vi "RSZVB Get Generator Attenuator Mode.vi"(8 "error in (no error)":errorcluster {"code" format="%.0x"}, 9 "Port (1)":i32=1, 10 "Channel (1)":i32=1, 11 "VISA session":refnum<visa-resource-name>) -> (0 "error out":errorcluster {"code" format="%.0x"}, 1 "Attenuation Mode":i32, 3 "dup VISA session":refnum<visa-resource-name>)   [LabVIEW 2011]
doc: "This VI returns the mode of the attenuation factor for the generated wave at test port no. <Pt>. \n\nNote(s):\n\n(1) This VI can be used only with R&S ZVA and ZVB instruments.\n\nRemote-control command(s):\nSOURce<Ch>:POWer<Pt>:ATTenuation:MODE?"
uses:
  _utility/RSZVB Global Data.vi
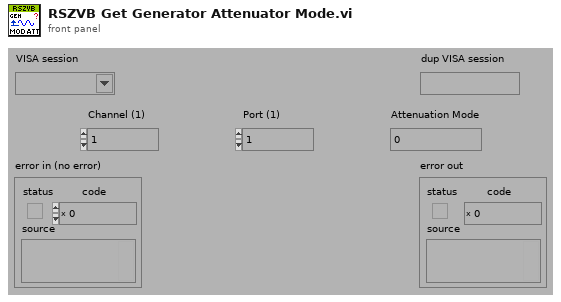
[diagram p1: front panel]
types:
  T1 = cluster{"Error Checking (T: On)":bool, "Installed Options":string[], "Data Valid?":bool, "Ports":i32, "Model":string[], "Option Checking (T: On)":bool}[]
  T2 = cluster{"Error Checking (T: On)":bool, "Installed Options":string[], "Data Valid?":bool, "Ports":i32, "Model":string[], "Option Checking (T: On)":bool}
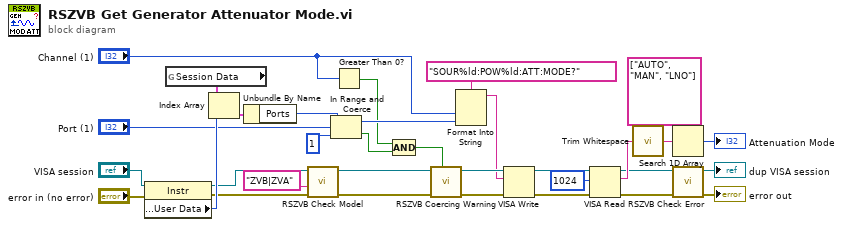
[diagram p0: block diagram]
diagram:
  n1 = property class="Instr"(reference="VISA session", error in="error in (no error)") -> (reference out=w23:refnum<visa-resource-name>, error out=w24:errorcluster, "General Settings:User Data"=w25:u32)
  n2 = global read "RSZVB Global Data.vi" "Session Data"() -> (w21:T1)
  n3 = Index Array(array=w21, index=w25) -> (element=w26:T2)
  n4 = Unbundle By Name(w26) -> ("Ports"=w22:i32)
  n5 = call "RSZVB Check Model.vi"("error in (no error)"=w24, "Model"="ZVB|ZVA" ("Options"), "VISA session"=w23) -> ("error out"=w29:errorcluster, "dup VISA session"=w28:refnum<visa-resource-name>)  [unwired: 7 in]
  n6 = In Range and Coerce(upper limit=w22, x="Port (1)", lower limit=1) -> (coerced(x)=w20:i32, In Range?=w18:bool)
  n7 = Greater Than 0?(x="Channel (1)") -> (x > 0?=w17:bool)
  n8 = Compound Arithmetic op=AND(w17, w18) -> (w16:bool)
  n9 = call "RSZVB Coercing Warning.vi"("In Range?"=w16, "error in (no error)"=w29, "VISA session"=w28) -> ("error out"=w31:errorcluster, "dup VISA session"=w32:refnum<visa-resource-name>)  [unwired: 7 in]
  n10 = Format Into String(format string="SOUR%ld:POW%ld:ATT:MODE?", "Channel (1)", w20) -> (resulting string=w30:string)  [unwired: 2 in, 1 out]
  n11 = VISA Write(VISA resource name=w32, write buffer=w30, error in (no error)=w31) -> (VISA resource name out=w5:refnum<visa-resource-name>, error out=w6:errorcluster)  [unwired: 1 out]
  n12 = VISA Read(VISA resource name=w5, byte count=u32 1024 ("byte count (0)"), error in (no error)=w6) -> (VISA resource name out=w3:refnum<visa-resource-name>, read buffer=w8:string, error out=w4:errorcluster)  [unwired: 1 out]
  n13 = call <vilib>:"Trim Whitespace.vi"("string"=w8) -> ("trimmed string"=w9:string)  [unwired: 1 in]
  n14 = Search 1D Array(1D array=string[] ["AUTO", "MAN", "LNO"], element=w9) -> (index of element=→"Attenuation Mode":i32)  [unwired: 1 in]
  n15 = call "RSZVB Check Error.vi"("error in (no error)"=w4, "VISA session"=w3) -> ("error out"=→"error out":errorcluster, "dup VISA session"=→"dup VISA session":refnum<visa-resource-name>)  [unwired: 8 in]
